vi "RX Message.vi"(8 "error in (no error)":errorcluster, 11 "VIN in":refnum<class "VIN.lvclass">) -> (0 "error out":errorcluster, 2 "String":string, 3 "VIN out":refnum<class "VIN.lvclass">)   [LabVIEW 2011, in "VIN.lvclass"]
uses:
  VIN.lvclass
  PID.lvclass
  <userlib>/Bloomy Controls/Timing/BCI_Timing.lvlib
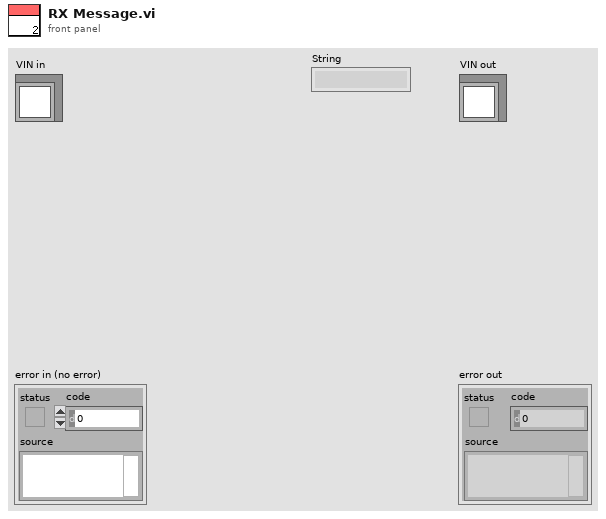
[diagram p1: front panel]
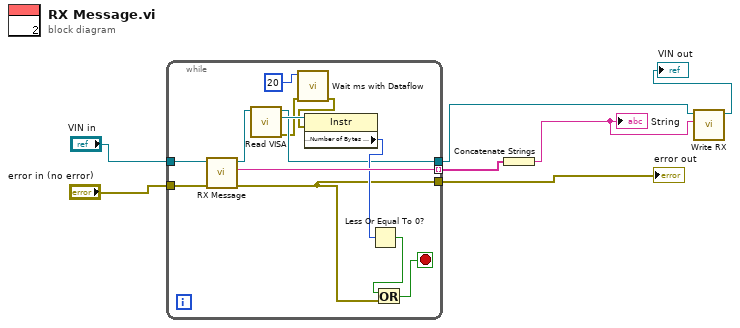
[diagram p0: block diagram]
diagram:
  n1 = while {
    tunnel: [w11] -> w7
    tunnel: [w20] -> w4 mode=indexing
    tunnel: "error in (no error)" -> [w19]
    tunnel: "VIN in" -> [w18]
    tunnel: [w14] -> w3
    stop <- w12 stop-if-true
    n2 = call-parent "RX Message.vi"("error in (no error)"=w19, "PID in"=w18) -> ("error out"=w11:errorcluster, "String"=w20:string, "PID out"=w15:refnum<class "VIN.lvclass">)  [unwired: 7 in]
    n3 = call "Read VISA.vi"("PID in"=w15) -> ("error out"=w10:errorcluster, "VISA"=w17:refnum<visa-resource-name>, "PID out"=w14:refnum<class "VIN.lvclass">)  [unwired: 8 in]
    n4 = call <userlib>:"Wait ms with Dataflow.vi"("error in (no error)"=w10, "milliseconds to wait"=u32 20) -> ("error out"=w9:errorcluster)  [unwired: 8 in, 1 out]
    n5 = property class="Instr"(reference=w17, error in=w9) -> ("Serial Settings:Number of Bytes at Serial Port"=w16:u32)  [unwired: 2 out]
    n6 = Less Or Equal To 0?(x=w16) -> (x <= 0?=w13:bool)
    n7 = Or(x=w13, y=w11) -> (x .or. y?=w12:bool)
  }
  "error out" <- w7
  n8 = Concatenate Strings(w4) -> (w1:string)
  "String" <- w1
  n9 = call "Write RX.vi"("RX"=w1, "PID in"=w3) -> ("PID out"=→"VIN out":refnum<class "VIN.lvclass">)  [unwired: 8 in, 1 out]
